vi "Room API Test.vi"() -> ()   [LabVIEW 2015]
uses:
  NurseStation/TypeDef/SelectedRoom.ctl
  LVClasses/Flags/ColorFlags.ctl
  LVRestAPI/TypeDef/FGVAction.ctl
  LVRestAPI/RoomRestApi.lvlib
  LVClasses/Room/Room.lvclass
  LVClasses/Flags/Flags.lvclass
panel:
  in  "Flags":bool[](array[boolean])
  in  "Request":string
  in  "Personnel":string
  out "Response":string
  out "Error Out":errorcluster
  out "Selected Room":T1={"Room Number"=0, "RoomNumFlags"={"Flag State"=[1, 3, 5, 7]}, "BedVacant"=FALSE, "InRoomPersonnel"=[], "RoomRequests"=[]}
  in  "Refresh Button":bool
  in  "Room":i32
  in  "Remove Request":bool
  in  "Add Request":bool
  in  "Remove Personnel":bool
  in  "Add Personnel":bool
  in  "stop":bool
  in  "URL":string="http://127.0.0.1:8001/RivERWebService/"
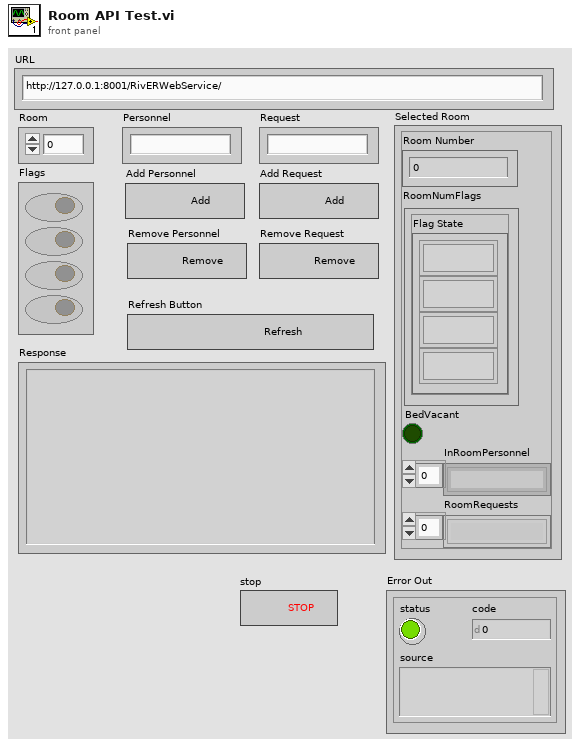
[diagram p1: front panel]
types:
  T1 = typedef "SelectedRoom.ctl" = cluster{"Room Number":u8, "RoomNumFlags":T2, "BedVacant":bool, "InRoomPersonnel":string[], "RoomRequests":string[]}
  T2 = typedef "Flags.lvclass/ColorFlags.ctl" = cluster{"Flag State":u8[]}
  T3 = typedef "FGVAction.ctl" = enum16{"Get", "Set"}
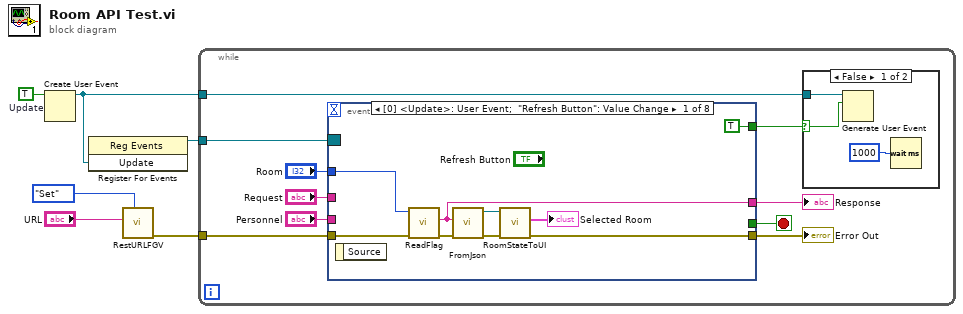
[diagram p0: block diagram]
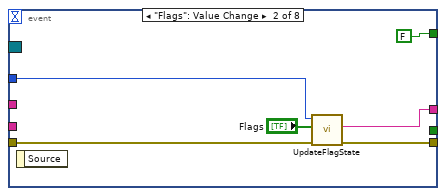
[diagram p3: hidden frame]
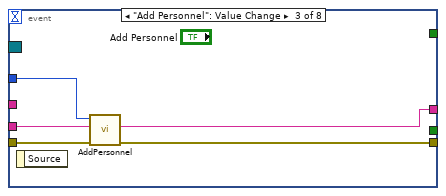
[diagram p4: hidden frame]
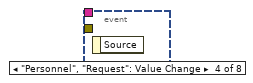
[diagram p5: hidden frame]
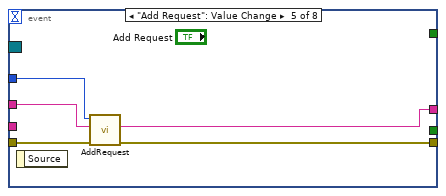
[diagram p6: hidden frame]
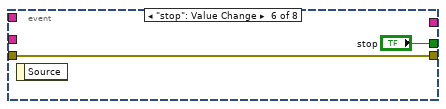
[diagram p7: hidden frame]
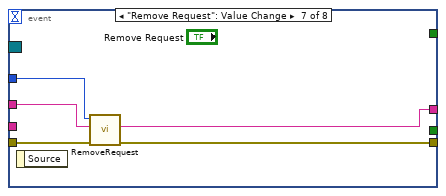
[diagram p8: hidden frame]
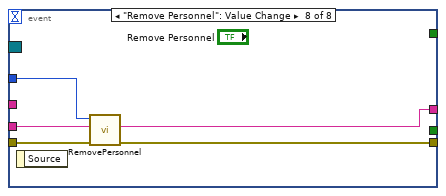
[diagram p9: hidden frame]
diagram:
  w3 = TRUE  # Update
  n1 = Create User Event(user event datatype=w3) -> (user event=w2:refnum<user-event>)  [unwired: 1 in, 1 out]
  n2 = register-events(w2) -> (reference out=w1:refnum<event-registration>)  [unwired: 2 in, 1 out]
  n3 = call "RestURLFGV.vi"("Action"=FGVAction."Set", "URL"="URL") -> ("error out"=w4:errorcluster)  [unwired: 8 in, 1 out]
  n4 = while {
    tunnel: w4 -> [w15]
    tunnel: w2 -> [w8]
    tunnel: w1 -> [w7]
    stop <- w10 stop-if-true
    n5 = event shown="[0] <Update>: User Event;  \"Refresh Button\": Value Change" {
      selector: w7 -> [_ _ _ _ _ _ _ _]
      dyn-events: _ -> [_ _ _ _ _ _ _ _]
      timeout: _ -> [_ _ _ _ _ _ _ _]
      tunnel: "Room" -> [w28 w33 w39 _ w44 _ w51 w56]
      tunnel: w15 -> [w25 w30 w37 _ w41 w45 w49 w53]
      tunnel: [w22 w31 w36 _ w40 w45 w48 w52] -> w14
      tunnel: "Personnel" -> [_ _ w38 _ _ _ _ w55]
      tunnel: [w21 w32 w35 _ w42 _ w47 w54] -> w13
      tunnel: "Request" -> [_ _ _ _ w43 _ w50 _]
      tunnel: [_ _ _ _ _ "stop" _ _] -> w10
      tunnel: [TRUE FALSE _ _ _ _ _ _] -> w9
      event User Event; "Refresh Button": Value Change {
        n6 = event-data() -> ()  [unwired: 1 in, 1 out]
        n7 = call "ReadFlag.vi"("error in (no error)"=w25, "Room Number"=w28) -> ("error out"=w24:errorcluster, "Flags JSON"=w21:string)  [unwired: 8 in]
        n8 = call "FromJson.vi"("error in (no error)"=w24, "String"=w21) -> ("error out"=w23:errorcluster, "Room out"=w27:refnum<class "Room.lvclass">)  [unwired: 8 in]
        n9 = call "RoomStateToUI.vi"("error in"=w23, "Room In"=w27) -> ("error out"=w22:errorcluster, "Selected Room"=→"Selected Room":T1)  [unwired: 7 in, 1 out]
      }
      event "Flags": Value Change {
        n10 = event-data() -> ()  [unwired: 1 in, 1 out]
        n11 = call "UpdateFlagState.vi"("error in (no error)"=w30, "FlagState"="Flags", "Room Number"=w33) -> ("error out"=w31:errorcluster, "Response"=w32:string)  [unwired: 7 in]
      }
      event "Add Personnel": Value Change {
        n12 = event-data() -> ()  [unwired: 1 in, 1 out]
        n13 = call "AddPersonnel.vi"("error in (no error)"=w37, "Personnel"=w38, "Room Number"=w39) -> ("error out"=w36:errorcluster, "Response"=w35:string)  [unwired: 7 in]
      }
      event "Personnel", "Request": Value Change {
        n14 = event-data() -> ()  [unwired: 1 in, 1 out]
      }
      event "Add Request": Value Change {
        n15 = event-data() -> ()  [unwired: 1 in, 1 out]
        n16 = call "AddRequest.vi"("error in (no error)"=w41, "Request"=w43, "Room Number"=w44) -> ("error out"=w40:errorcluster, "Response"=w42:string)  [unwired: 7 in]
      }
      event "stop": Value Change {
        n17 = event-data() -> ()  [unwired: 1 in, 1 out]
      }
      event "Remove Request": Value Change {
        n18 = event-data() -> ()  [unwired: 1 in, 1 out]
        n19 = call "RemoveRequest.vi"("error in (no error)"=w49, "Request"=w50, "Room Number"=w51) -> ("error out"=w48:errorcluster, "Response"=w47:string)  [unwired: 7 in]
      }
      event "Remove Personnel": Value Change {
        n20 = event-data() -> ()  [unwired: 1 in, 1 out]
        n21 = call "RemovePersonnel.vi"("error in (no error)"=w53, "Personnel"=w55, "Room Number"=w56) -> ("error out"=w52:errorcluster, "Response"=w54:string)  [unwired: 7 in]
      }
    }
    "Response" <- w13
    "Error Out" <- w14
    n22 = case shown="False" w9 {
      selector: w9 -> [w17 _]
      tunnel: w8 -> [w18 _]
      frame False {
        n23 = Generate User Event(user event=w18, event data cluster=w17) -> ()  [unwired: 2 in, 2 out]
        n24 = Wait (ms)(milliseconds to wait=u32 1000) -> ()  [unwired: 1 out]
      }
      frame True {
      }
    }
  }
